vi "attach subscriber.vi"(8 "error in":errorcluster, 10 "stream publisher":refnum<class "data bus stream subscriber.lvclass">, 11 "stream publisher in":refnum<class "data bus stream publisher.lvclass">) -> (0 "error out":errorcluster, 3 "stream publisher out":refnum<class "data bus stream publisher.lvclass">)   [LabVIEW 2013, in "data bus stream publisher.lvclass"]
uses:
  data bus stream publisher.lvclass
  subscriber/data bus stream subscriber.lvclass
  data bus stream publisher.lvclass/data bus stream publisher.ctl
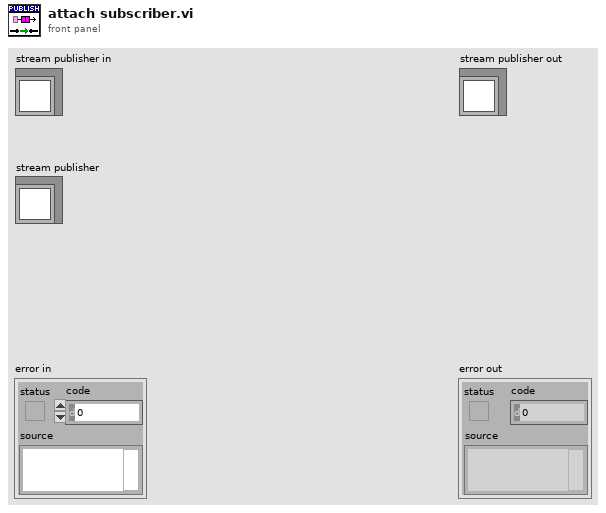
[diagram p1: front panel]
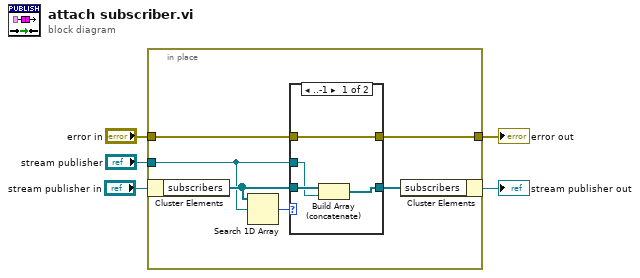
[diagram p0: block diagram]
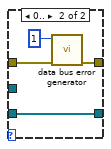
[diagram p2: hidden frame]
diagram:
  n1 = in-place {
    in-place-border: "stream publisher" -> [w6]
    in-place-border: "error in" -> [w10]
    in-place-border: [w9] -> w1
    n2 = in-place-cluster #1("stream publisher in") -> ("subscribers"=w7:refnum<class "data bus stream subscriber.lvclass">[])
    n3 = Search 1D Array(1D array=w7, element=w6) -> (index of element=w11:i32)  [unwired: 1 in]
    n4 = case shown="..-1" w11 {
      tunnel: w10 -> [w13 w19]
      tunnel: [w13 w18] -> w9
      tunnel: [w14 w16] -> w8
      tunnel: w7 -> [w15 w16]
      tunnel: w6 -> [w12 _]
      frame ..-1 {
        n5 = Build Array (concatenate)(w15, w12) -> (w14:refnum<class "data bus stream subscriber.lvclass">[])
      }
      frame 0.. {
        n6 = call "data bus error generator.vi"("error in"=w19, "error code (0)"=1) -> ("error out"=w18:errorcluster)  [unwired: 7 in]
      }
    }
    n7 = in-place-cluster #1("subscribers"=w8) -> (→"stream publisher out":refnum<class "data bus stream publisher.lvclass">)
  }
  "error out" <- w1
